vi "Test New Node.vi"(8 "error in (no error)":errorcluster) -> (0 "error out":errorcluster)   [LabVIEW 2017, in "Unit Tests.lvlib"]
uses:
  Unit Tests.lvlib
  source/Browser Core/Server Classes/Base Tree/Base Tree.lvclass
  source/Browser Core/Node Classes/Generic Node/Generic Node.lvclass/Generic Node.ctl
  <vilib>/addons/_JKI Toolkits/Caraya/classes/Test/Test.lvclass
  source/Browser Core/Node Classes/Generic Node/Generic Node.lvclass
  <vilib>/addons/_JKI Toolkits/Caraya/classes/Assert/Assert.lvclass
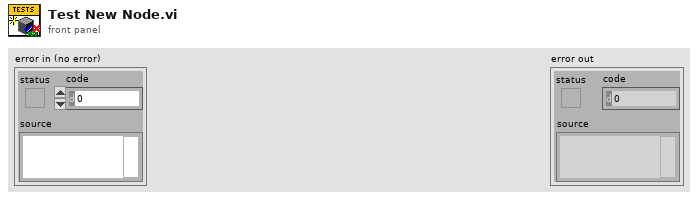
[diagram p1: front panel]
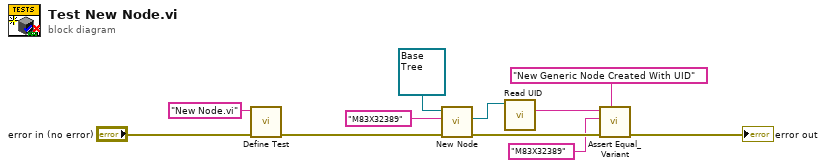
[diagram p0: block diagram]
diagram:
  n1 = call <vilib>:"Define Test.vi"("error in (no error)"="error in (no error)", "Label (VI Title)"="New Node.vi") -> ("error out"=w8:errorcluster)  [unwired: 9 in]
  n2 = call-dynamic "New Node.vi"("error in (no error)"=w8, "UID"="M83X32389", "Base Tree in"=refnum<class "Base Tree.lvclass"> refnum) -> ("error out"=w6:errorcluster, "Generic Node out"=w7:refnum<class "Generic Node.lvclass">)  [unwired: 6 in, 1 out]
  n3 = call "Read UID.vi"("Generic Node in"=w7) -> ("UID"=w5:string)  [unwired: 8 in, 2 out]
  n4 = call <vilib>:"Assert Equal_Variant.vi"("Label"="New Generic Node Created With UID", "error in (no error)"=w6, "Y"="M83X32389" ("UID"), "X"=w5) -> ("error out"=→"error out":errorcluster)  [unwired: 7 in]
